vi "SetT0.vi"(8 "error in (no error)":errorcluster, 11 "waveform":waveform(dbl)) -> (0 "error out":errorcluster, 3 "output waveform":waveform(dbl))   [LabVIEW 2017]
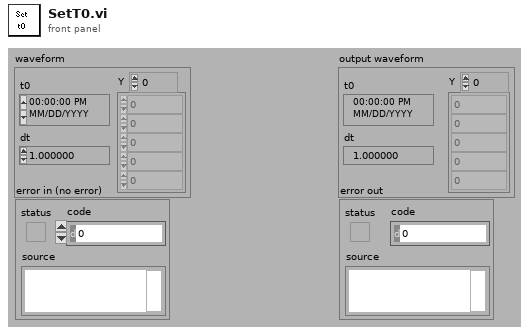
[diagram p1: front panel]
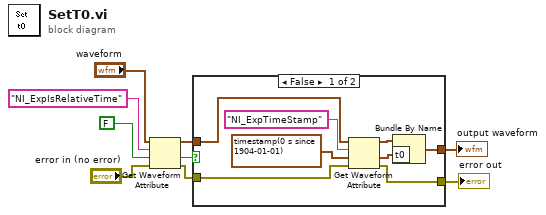
[diagram p0: block diagram]
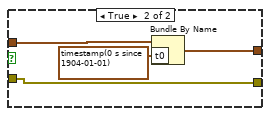
[diagram p2: hidden frame]
diagram:
  n1 = Get Waveform Attribute(4:"error in (no error)", 5:FALSE, 6:"NI_ExpIsRelativeTime" ("name"), 7:"waveform") -> (0:w3:errorcluster, 1:w4:bool, 3:w7:waveform(dbl))  [unwired: 1 out]
  n2 = case shown="False" w4 {
    tunnel: [w17 w20] -> w9
    tunnel: w7 -> [w14 w19]
    tunnel: w3 -> [w11 w18]
    tunnel: [w10 w18] -> w2
    frame False {
      n3 = Get Waveform Attribute(4:w11, 5:timestamp(0 s since 1904-01-01), 6:"NI_ExpTimeStamp" ("name"), 7:w14) -> (0:w10:errorcluster, 1:w12:timestamp, 3:w13:waveform(dbl))  [unwired: 1 out]
      n4 = Bundle By Name(cluster=w13, "t0"=w12) -> (w17:waveform(dbl))
    }
    frame True {
      n5 = Bundle By Name(cluster=w19, "t0"=timestamp(0 s since 1904-01-01)) -> (w20:waveform(dbl))
    }
  }
  "output waveform" <- w9
  "error out" <- w2
